vi "auto_ctrl_bypass_valve.vi"(4 "ref_reinit":refnum<vi>, 6 "ref_sp_turn":refnum<vi>, 7 "time_last_ctrl_in":timestamp, 8 "turn_org":dbl=0.8 format="%.1f", 9 "level_set":dbl=80.0 format="%.1f", 10 "enable_auto_ctrl":bool caption="Auto Control", 11 "level":dbl=90.0 format="%.1f") -> (0 "turn_new":dbl format="%.3f", 1 "status":u32(colorbox), 5 "time_last_ctrl_out":timestamp)   [LabVIEW 2019]
doc: "This example demonstrates how to simulate a general PID controller."
uses:
  <vilib>/addons/control/pid/pid.llb/PID (DBL).vi
  <vilib>/addons/control/pid/NI_PID_pid.lvlib
panel:
  in  "turn_max":dbl=1.2 format="%.1f"
  in  "turn_min":dbl=0.2 format="%.1f"
  out "MV":dbl format="%.1f"
  in  "ctrl_interval":dbl=5.0
  in  "PID Range":cluster{"High":dbl, "Low":dbl}={"High"=20.0, "Low"=-20.0} {"Low" format="%.1f"; "High" format="%.1f"}
  in  "PID gains":T1={"proportional gain (Kc)"=0.2, "integral time (Ti, min)"=2.0, "derivative time (Td, min)"=0.2} {"derivative time (Td, min)" format="%.4f"; "integral time (Ti, min)" format="%.4f"; "proportional gain (Kc)" format="%.3f"}
  # "sec"
  # "gain = delta_turn / delta_level ~ 0.1 / 1 = 0.1"
  # "turn"
  # "turn"
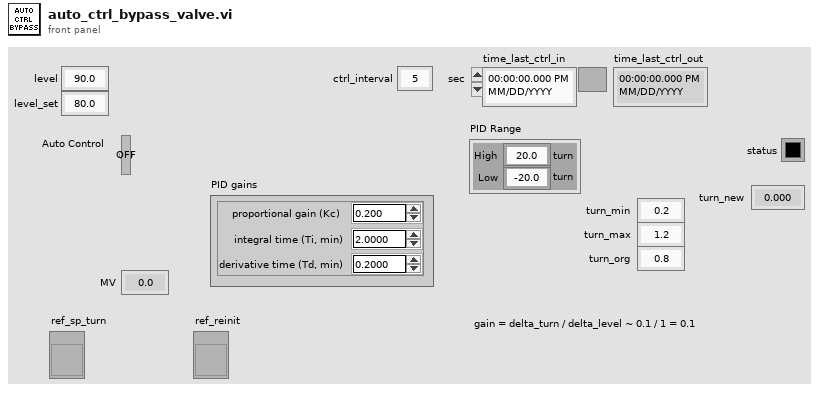
[diagram p1: front panel]
types:
  T1 = cluster{"proportional gain (Kc)":dbl, "integral time (Ti, min)":dbl, "derivative time (Td, min)":dbl}
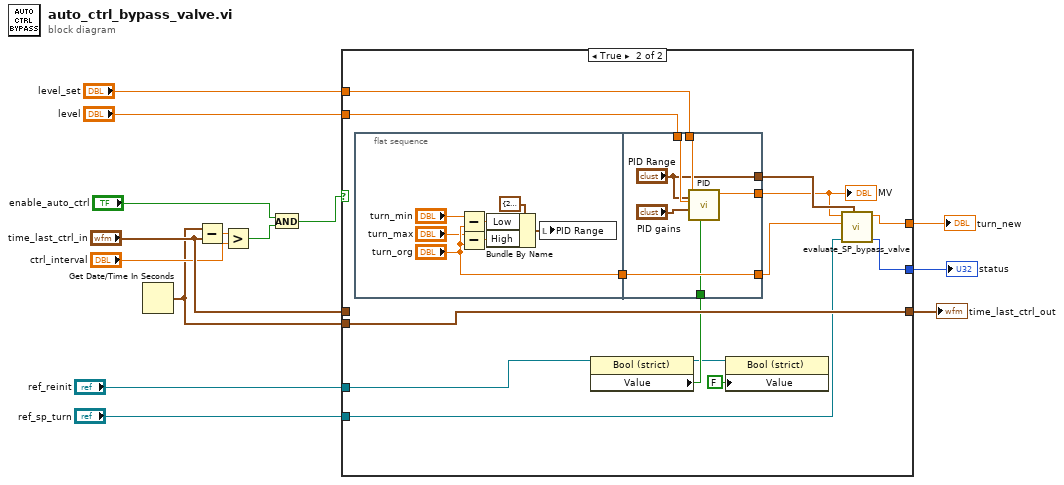
[diagram p0: block diagram]
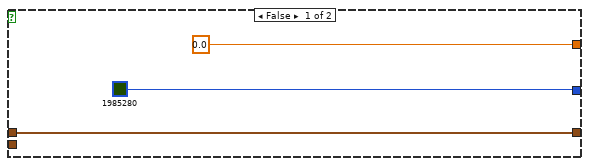
[diagram p2: hidden frame]
diagram:
  n1 = Get Date/Time In Seconds() -> (seconds since 1Jan1904=w4:timestamp)
  n2 = Subtract(x=w4, y="time_last_ctrl_in") -> (x-y=w5:dbl)
  n3 = Greater?(x=w5, y="ctrl_interval") -> (0:w3:bool)
  n4 = And(x="enable_auto_ctrl", y=w3) -> (x .and. y?=w1:bool)
  n5 = case shown="True" w1 {
    tunnel: [0.0 ("F_O_new") w28] -> w14
    tunnel: [u32 1985280 ("alarm_status") w31] -> w13
    tunnel: "level_set" -> [_ w24]
    tunnel: "level" -> [_ w25]
    tunnel: "ref_sp_turn" -> [_ w29]
    tunnel: [w16 w30] -> w7
    tunnel: w4 -> [_ w30]
    tunnel: "time_last_ctrl_in" -> [w16 _]
    tunnel: "ref_reinit" -> [_ w21]
    frame False {
    }
    frame True {
      n6 = flat-sequence {
        tunnel: ["turn_org"] -> w26
        tunnel: [w45] -> w27
        tunnel: w26 -> [w45]
        tunnel: w25 -> [w43]
        tunnel: w24 -> [w42]
        tunnel: ["PID Range"] -> w23
        tunnel: [w40] -> w22
        tunnel: w20 -> [w39]
        frame #0 {
          n7 = Subtract(x="turn_min", y="turn_org") -> (x-y=w35:dbl)
          n8 = Subtract(x="turn_max", y="turn_org") -> (x-y=w36:dbl)
          n9 = Bundle By Name(cluster=cluster{"High":dbl, "Low":dbl} {"High"=20.0, "Low"=-20.0} ("PID Range"), "Low"=w35, "High"=w36) -> (w38:cluster{"High":dbl, "Low":dbl})
          n10 = local write "PID Range"(w38) -> ()
        }
        frame #1 {
          n11 = call-poly <vilib>:"PID.vi"("reinitialize? (F)"=w39, "output range"="PID Range", "PID gains"="PID gains", "process variable"=w43, "setpoint"=w42) -> ("output"=w40:dbl)  [unwired: 5 in, 1 out]
        }
      }
      n12 = property class="Bool (strict)"(reference=w21) -> (reference out=w19:refnum<vi>, "Value"=w20:bool)  [unwired: 1 in, 1 out]
      n13 = property class="Bool (strict)"(reference=w19, "Value"=FALSE) -> ()  [unwired: 1 in, 2 out]
      n14 = call "evaluate_SP_bypass_valve.vi"("PID Range"=w23, "ref_sp_ch1"=w29, "F_org"=w27, "control"=w22) -> ("status"=w31:u32, "F_new"=w28:dbl)  [unwired: 6 in]
      "MV" <- w22
    }
  }
  "turn_new" <- w14
  "status" <- w13
  "time_last_ctrl_out" <- w7
